vi "Set Log File Properties.vi"(8 "error in (no error)":errorcluster, 10 "Logger Parameters":T1, 11 "Refnum in":refnum<k34>) -> (0 "error out":errorcluster, 3 "Refnum out":refnum<k34>)   [LabVIEW 2019, in "Telemetry Engine.lvlib"]
uses:
  Types/Logger Data.ctl
  Types/Async Logger State Data.ctl
  Types/System Channels.ctl
  Types/Target Info.ctl
  Shared/Constants.vi
  Telemetry Engine.lvlib
  Shared/Telemetry Shared.lvlib
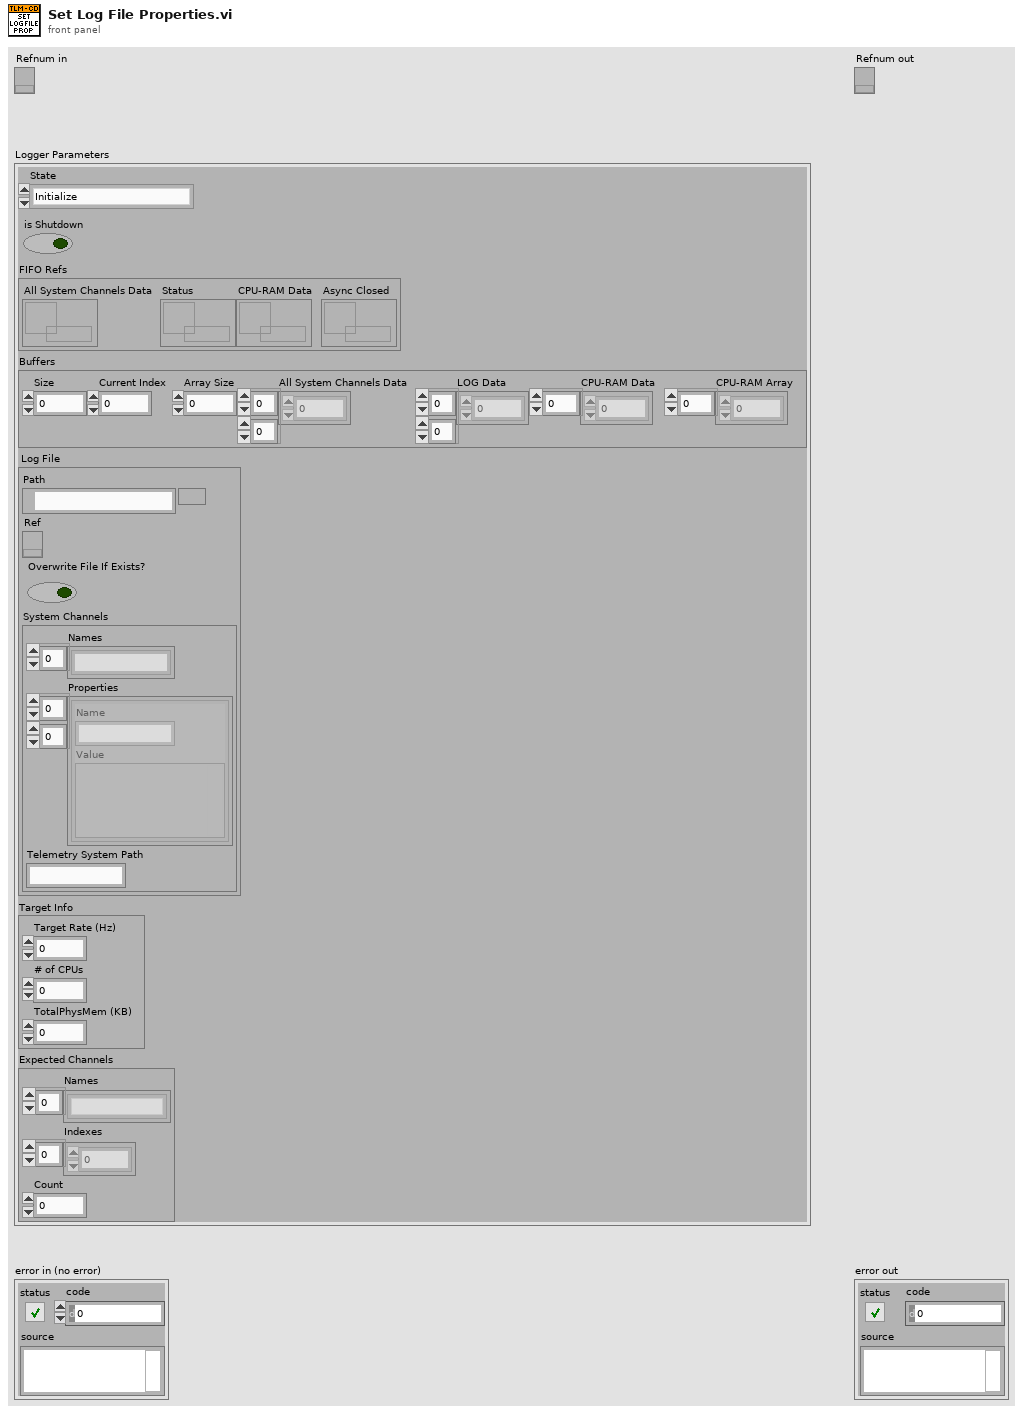
[diagram p1: front panel]
types:
  T1 = typedef "Telemetry Engine.lvlib/Logger Data.ctl" = cluster{"State":T2, "is Shutdown":bool, "FIFO Refs":cluster{"All System Channels Data":refnum<k33>, "Status":refnum<k33>, "CPU-RAM Data":refnum<k33>, "Async Closed":refnum<k33>}, "Buffers":cluster{"Size":i32, "Current Index":i32, "Array Size":i32, "All System Channels Data":dbl[][], "LOG Data":dbl[][], "CPU-RAM Data":dbl[], "CPU-RAM Array":dbl[]}, "Log File":cluster{"Path":path, "Ref":refnum<k34>, "Overwrite File If Exists?":bool, "System Channels":T3}, "Target Info":T4, "Expected Channels":cluster{"Names":string[], "Indexes":i32[], "Count":i32}}
  T2 = typedef "Telemetry Engine.lvlib/Async Logger State Data.ctl" = enum16{"Initialize", "Read System Channels FIFO", "Filter System Channels", "Read CPU-RAM FIFO", "Log Data", "Shutdown"}
  T3 = typedef "Telemetry Engine.lvlib/System Channels.ctl" = cluster{"Names":string[], "Properties":cluster{"Name":string, "Value":variant}[][], "Telemetry System Path":string}
  T4 = typedef "Telemetry Engine.lvlib/Target Info.ctl" = cluster{"Target Rate (Hz)":dbl, "# of CPUs":u32, "TotalPhysMem (KB)":dbl}
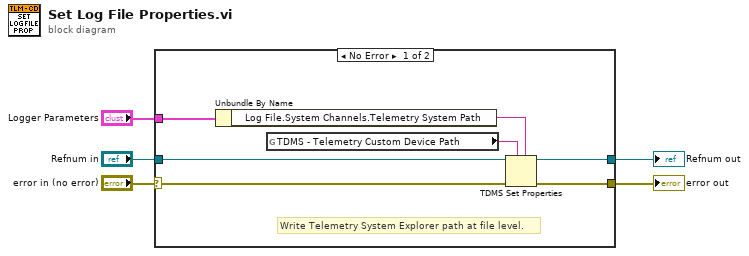
[diagram p0: block diagram]
diagram:
  n1 = case shown="No Error" "error in (no error)" {
    selector: "error in (no error)" -> [w11 w14]
    tunnel: "Logger Parameters" -> [w6 _]
    tunnel: "Refnum in" -> [w12 w13]
    tunnel: [w9 w13] -> w4
    tunnel: [w10 w14] -> w3
    frame No Error {
      # "Write Telemetry System Explorer path at file level."
      n2 = Unbundle By Name(w6) -> ("Log File.System Channels.Telemetry System Path"=w8:string)
      n3 = global read "Constants.vi" "TDMS - Telemetry Custom Device Path"() -> (w7:string)
      n4 = TDMS Set Properties(5:w8, 7:w7, 8:w11, 11:w12) -> (0:w10:errorcluster, 3:w9:refnum<k34>)  [unwired: 2 in, 2 out]
    }
    frame Error {
    }
  }
  "Refnum out" <- w4
  "error out" <- w3
